vi "Drive to Line.vi"(7 "Description":string, 8 "Command Info In":T1, 10 "Target Angle":dbl, 11 "Distance":dbl) -> (0 "Command Info Out":T1)   [LabVIEW 2018]
doc: "This VI notifies the subsystem to the new setpoint."
uses:
  <vilib>/Rock Robotics/WPI/Framework/Command Status Info.ctl
  <vilib>/Rock Robotics/WPI/Framework/Completion Status.ctl
  <vilib>/Rock Robotics/WPI/Framework/Completion Notifier.ctl
  Implementation/Drive Setpoints.ctl
  Implementation/Drive Operations.ctl
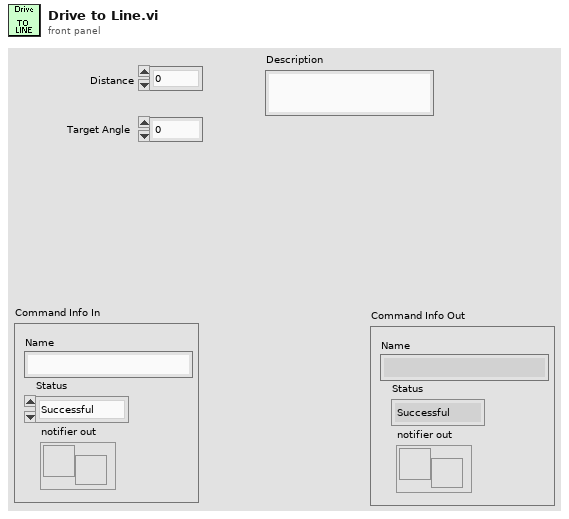
[diagram p1: front panel]
types:
  T1 = typedef "Command Status Info.ctl" = cluster{"Name":string, "Status":T2, "notifier out":T3}
  T2 = typedef "Completion Status.ctl" = enum16{"Successful", "Aborted", "Incomplete"}
  T3 = typedef "Completion Notifier.ctl" = refnum<notifier>
  T4 = typedef "Drive Setpoints.ctl" = cluster{"Operation":T5, "Left Setpoint":dbl, "Right Setpoint":dbl, "Duration":dbl, "Distance":dbl, "Target Angle":dbl, "Speed":dbl}
  T5 = typedef "Drive Operations.ctl" = enum16{"Reserve", "Read Current", "Immediate", "Drive for Time", "Drive for Distance", "Drive Distance Line", "Drive to Angle Relative", "Drive to Angle", "Run Motion Profile", "Auto Turn", "Reset Encoders", "Reset Gyro"}
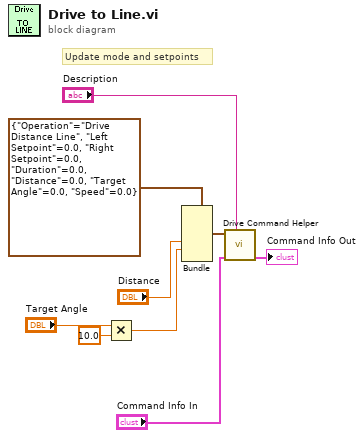
[diagram p0: block diagram]
diagram:
  # "Update mode and setpoints"
  n1 = Multiply(x="Target Angle", y=10.0) -> (x*y=w3:dbl)
  n2 = Bundle(cluster=T4 {"Operation"=enum."Drive Distance Line", "Left Setpoint"=0.0, "Right Setpoint"=0.0, "Duration"=0.0, "Distance"=0.0, "Target Angle"=0.0, "Speed"=0.0} ("SubSystem Data"), "Distance"="Distance", "Target Angle"=w3) -> (w5:T4)  [unwired: 5 in]
  n3 = call "Drive Command Helper.vi"("Description"="Description", "Command Info In"="Command Info In", "SubSystem Data"=w5) -> ("Command Info Out"=→"Command Info Out":T1)  [unwired: 6 in, 2 out]
